vi "Disable UI.vi"(8 "error in (no error)":errorcluster, 11 "Operator UI Actor in":refnum<class "Measurement UI.lvclass">) -> (0 "error out":errorcluster, 3 "Operator UI Actor out":refnum<class "Measurement UI.lvclass">)   [LabVIEW 2016, in "Measurement UI.lvlib" / "Measurement UI.lvclass"]
uses:
  Measurement UI.lvclass
  Measurement UI.lvclass/Measurement UI.ctl
  Accessors/Read Digitizer.vi
  Accessors/Read View Results.vi
  Accessors/Read Load New Measurement.vi
  Accessors/Read Function Generator.vi
  Read Multimeter.vi
  Accessors/Read Run.vi
  Accessors/Read Measurement.vi
  Accessors/Read Power Supply.vi
  Accessors/Read Show FP_.vi
  Accessors/Read Results Listbox.vi
  User Interface/UI.lvclass
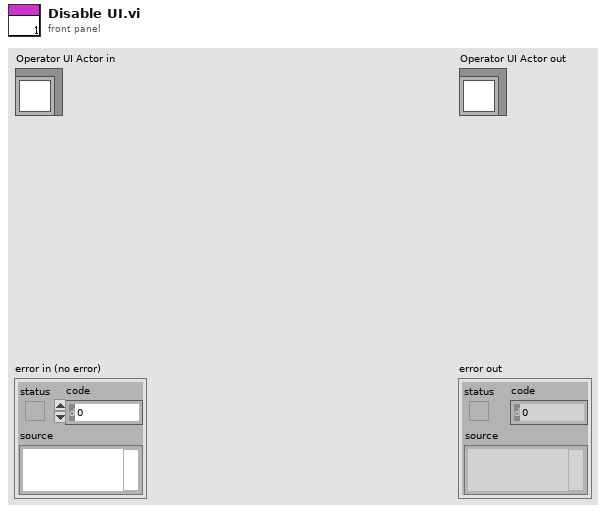
[diagram p1: front panel]
types:
  T1 = enum8{"Enabled", "Disabled", "Disabled and Grayed Out"}
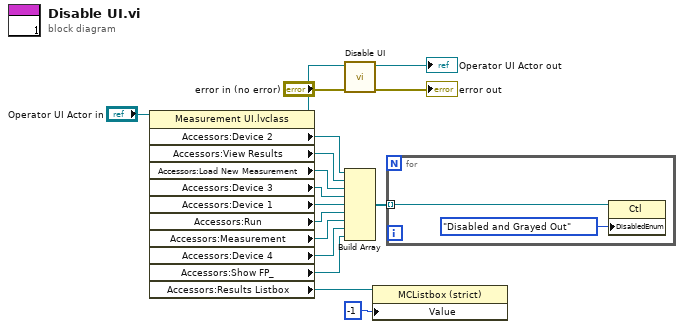
[diagram p0: block diagram]
diagram:
  n1 = property class="Measurement UI.lvclass"(reference="Operator UI Actor in") -> (reference out=w12:refnum<class "Measurement UI.lvclass">, "Accessors:Device 2"=w11:refnum<vi>, "Accessors:View Results"=w10:refnum<vi>, "Accessors:Load New Measurement"=w9:refnum<vi>, "Accessors:Device 3"=w8:refnum<vi>, "Accessors:Device 1"=w7:refnum<vi>, "Accessors:Run"=w6:refnum<vi>, "Accessors:Measurement"=w5:refnum<vi>, "Accessors:Device 4"=w4:refnum<vi>, "Accessors:Show FP_"=w3:refnum<vi>, "Accessors:Results Listbox"=w1:refnum<vi>)  [unwired: 1 in, 1 out]
  n2 = call-parent "Disable UI.vi"("error in (no error)"="error in (no error)", "UI in"=w12) -> ("error out"=→"error out":errorcluster, "UI out"=→"Operator UI Actor out":refnum<class "Measurement UI.lvclass">)  [unwired: 8 in]
  n3 = Build Array(w11, w10, w9, w8, w7, w6, w5, w4, w3) -> (w14:refnum<vi>[])
  n4 = property class="MCListbox (strict)"(reference=w1, "Value"=-1 ("Listbox")) -> ()  [unwired: 1 in, 2 out]
  n5 = for {
    tunnel: w14 -> [w19] mode=indexing
    n6 = property class="Ctl"(reference=w19, "DisabledEnum"=T1."Disabled and Grayed Out" ("Disabled")) -> ()  [unwired: 1 in, 2 out]
  }
